vi "get_DataCollection.vi"(8 "error in (no error)":errorcluster, 11 "ScanModeDL090923Scaffold in":refnum<class "ImagingModeDL090923Scaffold.lvclass">) -> (0 "error out":errorcluster, 1 "DataCollection adapter":refnum<class "GenericAdapter.lvclass">, 2 "DataCollection":refnum<class "GenericDataCollection.lvclass">, 3 "ScanModeDL090923Scaffold out":refnum<class "ImagingModeDL090923Scaffold.lvclass">, 4 "DataCollection specification":T1, 6 "adapter path":path)   [LabVIEW 2010, in "ImagingModeDL090923Scaffold.lvclass"]
uses:
  ImagingModeDL090923Scaffold.lvclass
  DataCollection/GenericDataCollection/GenericDataCollection/GenericDataCollection.lvclass
  Adapter/GenericAdapter/GenericAdapter/GenericAdapter.lvclass
  common/clusters/plugin_specification.ctl
  ImagingModeDL090923Scaffold.lvclass/ImagingModeDL090923Scaffold.ctl
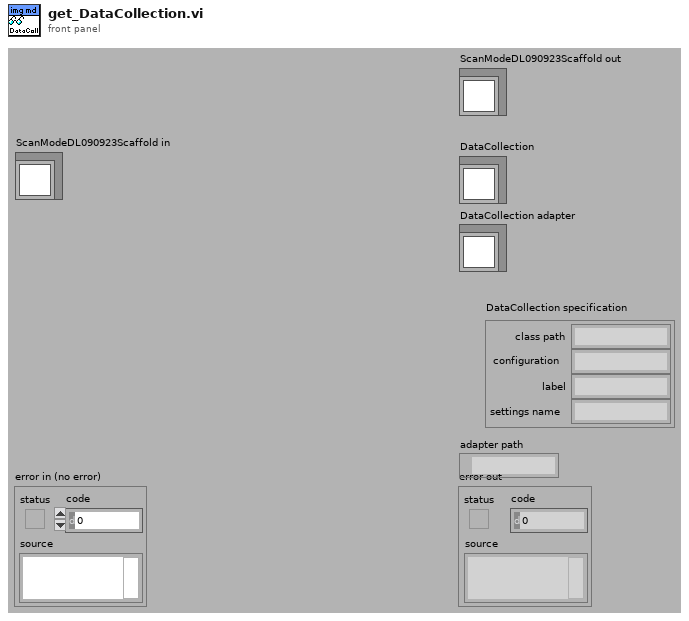
[diagram p1: front panel]
types:
  T1 = typedef "plugin_specification.ctl" = cluster{"class path":string, "configuration":string, "label":string, "settings name":string}
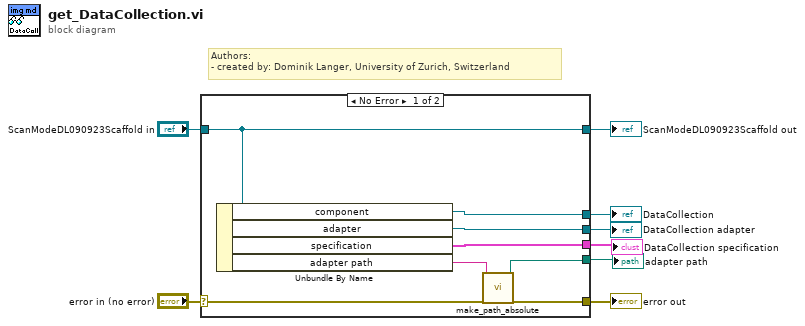
[diagram p0: block diagram]
diagram:
  # "Authors: \n- created by: Dominik Langer, University of Zurich, Switzerland"
  n1 = case shown="No Error" "error in (no error)" {
    selector: "error in (no error)" -> [w10 w17]
    tunnel: [w9 w17] -> w7
    tunnel: [w16 w18] -> w5
    tunnel: "ScanModeDL090923Scaffold in" -> [w16 w18]
    tunnel: [w15 _] -> w4
    tunnel: [w14 _] -> w3
    tunnel: [w13 _] -> w2
    tunnel: [w11 _] -> w1
    frame No Error {
      n2 = Unbundle By Name(w16) -> ("component"=w15:refnum<class "GenericDataCollection.lvclass">, "adapter"=w14:refnum<class "GenericAdapter.lvclass">, "specification"=w13:T1, "adapter path"=w12:string)
      n3 = call "make_path_absolute.vi"("error in (no error)"=w10, "relative path"=w12) -> ("error out"=w9:errorcluster, "absolute path"=w11:path)  [unwired: 8 in]
    }
    frame Error {
    }
  }
  "error out" <- w7
  "ScanModeDL090923Scaffold out" <- w5
  "DataCollection" <- w4
  "DataCollection adapter" <- w3
  "DataCollection specification" <- w2
  "adapter path" <- w1
